vi "Send Challenge Request.vi"(8 "error in (no error)":errorcluster, 11 "Connection in":refnum<class "Connection.lvclass">) -> (0 "error out":errorcluster, 1 "timeout":bool, 2 "Challenge Request":T1, 3 "Connection out":refnum<class "Connection.lvclass">)   [LabVIEW 2013, in "Connection_GOSPL.lvlib" / "Connection.lvclass"]
uses:
  Connection.lvclass
  challenge request -- cluster.ctl
  Connection.lvclass/Connection.ctl
  <vilib>/LabVIEW Open Source Project/Unicity/RandomStringGenerator/RandomStringGenerator.lvclass
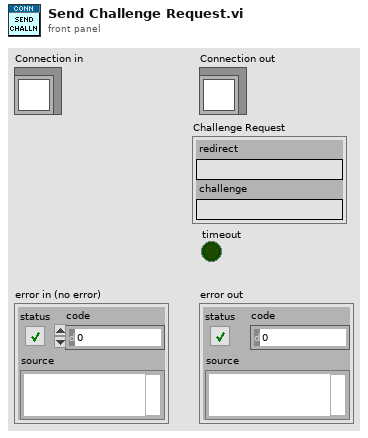
[diagram p1: front panel]
types:
  T1 = typedef "Connection_GOSPL.lvlib/Connection.lvclass/challenge request -- cluster.ctl" = cluster{"redirect":string, "challenge":string}
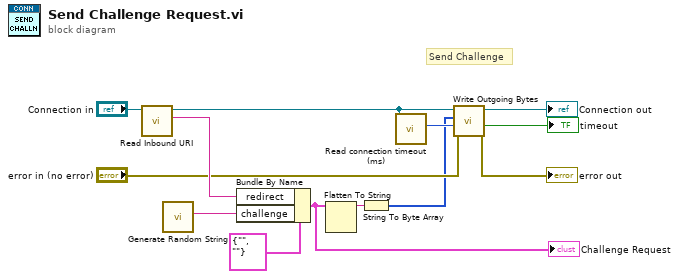
[diagram p0: block diagram]
diagram:
  # "Send Challenge"
  n1 = call "Read Inbound URI.vi"("Connection in"="Connection in") -> ("Inbound URI"=w13:string, "Connection out"=w4:refnum<class "Connection.lvclass">)  [unwired: 9 in]
  n2 = call <vilib>:"Generate Random String.vi"() -> ("Random String"=w7:string)  [unwired: 11 in]
  n3 = Bundle By Name(cluster=T1 {"redirect"="", "challenge"=""} ("Challenge"), "redirect"=w13, "challenge"=w7) -> (w1:T1)
  "Challenge Request" <- w1
  n4 = Flatten To String(anything=w1) -> (data string=w8:string)  [unwired: 3 in, 2 out]
  n5 = String To Byte Array(string=w8) -> (unsigned byte array=w9:u8[])
  n6 = call "Read connection timeout (ms).vi"("Connection in"=w4) -> ("connection timeout (ms)"=w10:i32)  [unwired: 8 in, 2 out]
  n7 = call-dynamic "Write Outgoing Bytes.vi"("error in (no error)"="error in (no error)", "timeout (2000 ms)"=w10, "Bytes"=w9, "Connection in"=w4) -> ("error out"=→"error out":errorcluster, "timeout"=→"timeout":bool, "Connection out"=→"Connection out":refnum<class "Connection.lvclass">)  [unwired: 5 in]
